vi "Send Email using SMTP Client Attachment.vi"(9 "Message 2":string="OPEN THE PIC BELOW", 10 "Subject 2":string="REAL TIME MONITORING", 11 "To: 2":string="pankaj7897@outlook.com") -> ()   [LabVIEW 2013]
doc: "Uses the SMTP Email Client to send an email to a standard or secure SMTP server."
uses:
  <vilib>/smtpClient/Set Message Text.vi
  <vilib>/smtpClient/LabVIEWSMTPClient.lvlib
panel:
  in  "Password 2":string="niyantra17"
  in  "Username 2":string="sass_niy135@hotmail.com"
  in  "Port 2":string="587"
  in  "Sender's Email Address 2":string="sass_niy135@hotmail.com"
  in  "Outgoing Mail Server (SMTP) 2":string="smtp.live.com"
  # "Outgoing Mail Server"
  # "Optional Parameters"
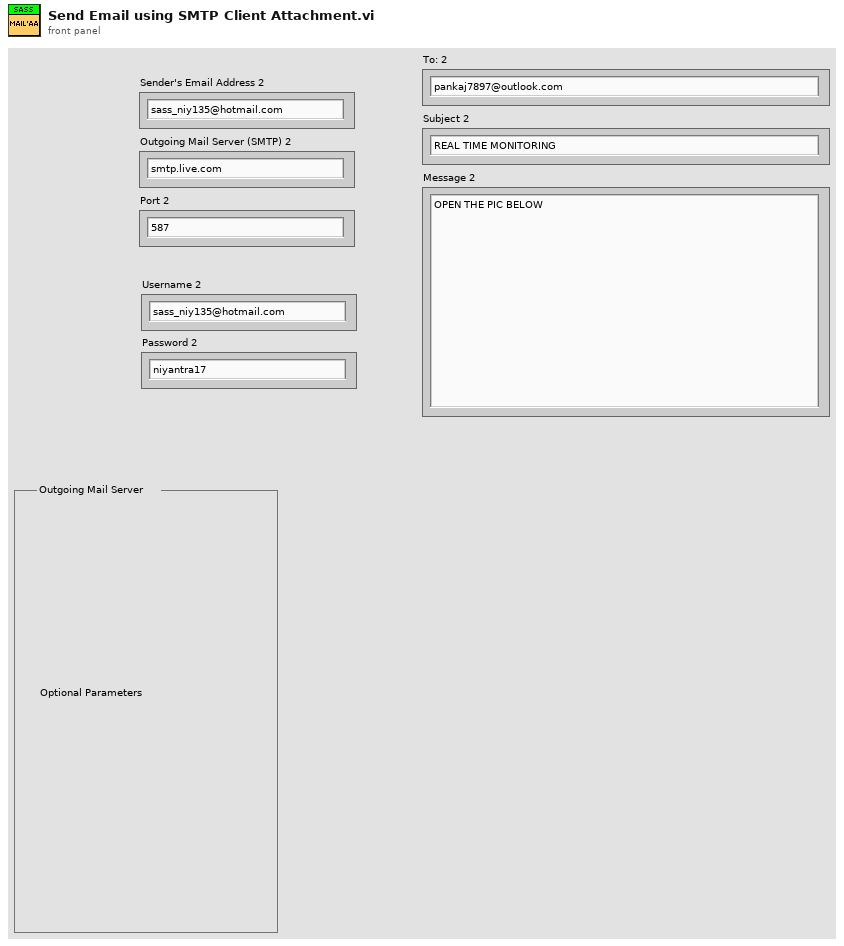
[diagram p1: front panel]
types:
  T1 = typedef "LabVIEWSMTPClient.lvlib/SmtpClientHandle.ctl" = refnum<k1>
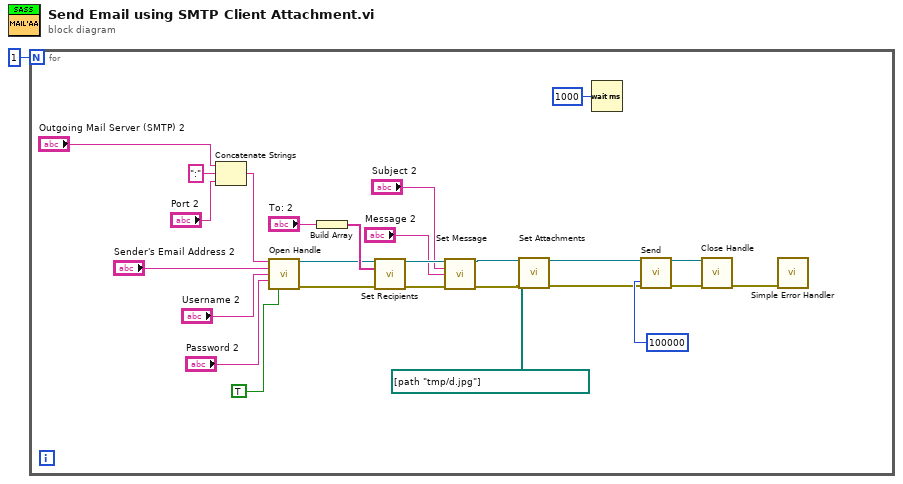
[diagram p0: block diagram]
diagram:
  n1 = for {
    N: 1 -> [_]
    n2 = Concatenate Strings("Outgoing Mail Server (SMTP) 2", ":" ("string"), "Port 2") -> (w24:string)
    n3 = call <vilib>:"Open Handle.vi"("server address"=w24, "from"="Sender's Email Address 2", "username"="Username 2", "password"="Password 2", "use TLS (false)"=TRUE) -> ("handle out"=w13:T1, "error out"=w12:errorcluster)  [unwired: 9 in]
    n4 = Build Array("To: 2") -> (w15:string[])
    n5 = call <vilib>:"Set Recipients.vi"("handle in"=w13, "to"=w15, "error in (no error)"=w12) -> ("handle out"=w19:T1, "error out"=w16:errorcluster)  [unwired: 11 in]
    n6 = call-poly <vilib>:"Set Message.vi"("handle in"=w19, "subject"="Subject 2", "plain text message"="Message 2", "error in (no error)"=w16) -> ("handle out"=w6:T1, "error out"=w5:errorcluster)  [unwired: 10 in]
    n7 = call <vilib>:"Set Attachments.vi"("handle in"=w6, "attachments"=path[] [path "tmp/d.jpg"], "error in (no error)"=w5) -> ("handle out"=w4:T1, "error out"=w3:errorcluster)  [unwired: 11 in]
    n8 = Wait (ms)(milliseconds to wait=u32 1000) -> ()  [unwired: 1 out]
    n9 = call <vilib>:"Send.vi"("handle in"=w4, "error in (no error)"=w3, "timeout in ms (10000)"=100000 ("timeout in ms")) -> ("handle out"=w11:T1, "error out"=w10:errorcluster)  [unwired: 10 in, 1 out]
    n10 = call <vilib>:"Close Handle.vi"("handle in"=w11, "error in (no error)"=w10) -> ("error out"=w8:errorcluster)  [unwired: 12 in, 1 out]
    n11 = call <vilib>:"Simple Error Handler.vi"("error in (no error)"=w8) -> ()  [unwired: 4 in, 5 out]
  }
